vi "FipsAdjacent.vi"() -> (11 "Fips":i32[](array[numeric]))   [LabVIEW 2017] (continued)
\"Perquimans County, NC\"\t37143\n\"Perquimans County, NC\"\t37143\t\"Tyrrell County, NC\"\t37177\n\"Perquimans County, NC\"\t37143\t\"Washington County, NC\"\t37187\n\"Person County, NC\"\t37145\t\"Caswell County, NC\"\t37033\n\"Person County, NC\"\t37145\t\"Durham County, NC\"\t37063\n\"Person County, NC\"\t37145\t\"Granville County, NC\"\t37077\n\"Person County, NC\"\t37145\t\"Orange County, NC\"\t37135\n\"Person County, NC\"\t37145\t\"Person County, NC\"\t37145\n\"Person County, NC\"\t37145\t\"Halifax County, VA\"\t51083\n\"Pitt County, NC\"\t37147\t\"Beaufort County, NC\"\t37013\n\"Pitt County, NC\"\t37147\t\"Craven County, NC\"\t37049\n\"Pitt County, NC\"\t37147\t\"Edgecombe County, NC\"\t37065\n\"Pitt County, NC\"\t37147\t\"Greene County, NC\"\t37079\n\"Pitt County, NC\"\t37147\t\"Lenoir County, NC\"\t37107\n\"Pitt County, NC\"\t37147\t\"Martin County, NC\"\t37117\n\"Pitt County, NC\"\t37147\t\"Pitt County, NC\"\t37147\n\"Pitt County, NC\"\t37147\t\"Wilson County, NC\"\t37195\n\"Polk County, NC\"\t37149\t\"Henderson County, NC\"\t37089\n\"Polk County, NC\"\t37149\t\"Polk County, NC\"\t37149\n\"Polk County, NC\"\t37149\t\"Rutherford County, NC\"\t37161\n\"Polk County, NC\"\t37149\t\"Greenville County, SC\"\t45045\n\"Polk County, NC\"\t37149\t\"Spartanburg County, SC\"\t45083\n\"Randolph County, NC\"\t37151\t\"Alamance County, NC\"\t37001\n\"Randolph County, NC\"\t37151\t\"Chatham County, NC\"\t37037\n\"Randolph County, NC\"\t37151\t\"Davidson County, NC\"\t37057\n\"Randolph County, NC\"\t37151\t\"Guilford County, NC\"\t37081\n\"Randolph County, NC\"\t37151\t\"Montgomery County, NC\"\t37123\n\"Randolph County, NC\"\t37151\t\"Moore County, NC\"\t37125\n\"Randolph County, NC\"\t37151\t\"Randolph County, NC\"\t37151\n\"Richmond County, NC\"\t37153\t\"Anson County, NC\"\t37007\n\"Richmond County, NC\"\t37153\t\"Hoke County, NC\"\t37093\n\"Richmond County, NC\"\t37153\t\"Montgomery County, NC\"\t37123\n\"Richmond County, NC\"\t37153\t\"Moore County, NC\"\t37125\n\"Richmond County, NC\"\t37153\t\"Richmond County, NC\"\t37153\n\"Richmond County, NC\"\t37153\t\"Scotland County, NC\"\t37165\n\"Richmond County, NC\"\t37153\t\"Stanly County, NC\"\t37167\n\"Richmond County, NC\"\t37153\t\"Chesterfield County, SC\"\t45025\n\"Richmond County, NC\"\t37153\t\"Marlboro County, SC\"\t45069\n\"Robeson County, NC\"\t37155\t\"Bladen County, NC\"\t37017\n\"Robeson County, NC\"\t37155\t\"Columbus County, NC\"\t37047\n\"Robeson County, NC\"\t37155\t\"Cumberland County, NC\"\t37051\n\"Robeson County, NC\"\t37155\t\"Hoke County, NC\"\t37093\n\"Robeson County, NC\"\t37155\t\"Robeson County, NC\"\t37155\n\"Robeson County, NC\"\t37155\t\"Scotland County, NC\"\t37165\n\"Robeson County, NC\"\t37155\t\"Dillon County, SC\"\t45033\n\"Robeson County, NC\"\t37155\t\"Horry County, SC\"\t45051\n\"Robeson County, NC\"\t37155\t\"Marlboro County, SC\"\t45069\n\"Rockingham County, NC\"\t37157\t\"Alamance County, NC\"\t37001\n\"Rockingham County, NC\"\t37157\t\"Caswell County, NC\"\t37033\n\"Rockingham County, NC\"\t37157\t\"Forsyth County, NC\"\t37067\n\"Rockingham County, NC\"\t37157\t\"Guilford County, NC\"\t37081\n\"Rockingham County, NC\"\t37157\t\"Rockingham County, NC\"\t37157\n\"Rockingham County, NC\"\t37157\t\"Stokes County, NC\"\t37169\n\"Rockingham County, NC\"\t37157\t\"Henry County, VA\"\t51089\n\"Rockingham County, NC\"\t37157\t\"Pittsylvania County, VA\"\t51143\n\"Rowan County, NC\"\t37159\t\"Cabarrus County, NC\"\t37025\n\"Rowan County, NC\"\t37159\t\"Davidson County, NC\"\t37057\n\"Rowan County, NC\"\t37159\t\"Davie County, NC\"\t37059\n\"Rowan County, NC\"\t37159\t\"Iredell County, NC\"\t37097\n\"Rowan County, NC\"\t37159\t\"Montgomery County, NC\"\t37123\n\"Rowan County, NC\"\t37159\t\"Rowan County, NC\"\t37159\n\"Rowan County, NC\"\t37159\t\"Stanly County, NC\"\t37167\n\"Rutherford County, NC\"\t37161\t\"Buncombe County, NC\"\t37021\n\"Rutherford County, NC\"\t37161\t\"Burke County, NC\"\t37023\n\"Rutherford County, NC\"\t37161\t\"Cleveland County, NC\"\t37045\n\"Rutherford County, NC\"\t37161\t\"Henderson County, NC\"\t37089\n\"Rutherford County, NC\"\t37161\t\"McDowell County, NC\"\t37111\n\"Rutherford County, NC\"\t37161\t\"Polk County, NC\"\t37149\n\"Rutherford County, NC\"\t37161\t\"Rutherford County, NC\"\t37161\n\"Rutherford County, NC\"\t37161\t\"Cherokee County, SC\"\t45021\n\"Rutherford County, NC\"\t37161\t\"Spartanburg County, SC\"\t45083\n\"Sampson County, NC\"\t37163\t\"Bladen County, NC\"\t37017\n\"Sampson County, NC\"\t37163\t\"Cumberland County, NC\"\t37051\n\"Sampson County, NC\"\t37163\t\"Duplin County, NC\"\t37061\n\"Sampson County, NC\"\t37163\t\"Harnett County, NC\"\t37085\n\"Sampson County, NC\"\t37163\t\"Johnston County, NC\"\t37101\n\"Sampson County, NC\"\t37163\t\"Pender County, NC\"\t37141\n\"Sampson County, NC\"\t37163\t\"Sampson County, NC\"\t37163\n\"Sampson County, NC\"\t37163\t\"Wayne County, NC\"\t37191\n\"Scotland County, NC\"\t37165\t\"Hoke County, NC\"\t37093\n\"Scotland County, NC\"\t37165\t\"Moore County, NC\"\t37125\n\"Scotland County, NC\"\t37165\t\"Richmond County, NC\"\t37153\n\"Scotland County, NC\"\t37165\t\"Robeson County, NC\"\t37155\n\"Scotland County, NC\"\t37165\t\"Scotland County, NC\"\t37165\n\"Scotland County, NC\"\t37165\t\"Marlboro County, SC\"\t45069\n\"Stanly County, NC\"\t37167\t\"Anson County, NC\"\t37007\n\"Stanly County, NC\"\t37167\t\"Cabarrus County, NC\"\t37025\n\"Stanly County, NC\"\t37167\t\"Davidson County, NC\"\t37057\n\"Stanly County, NC\"\t37167\t\"Montgomery County, NC\"\t37123\n\"Stanly County, NC\"\t37167\t\"Richmond County, NC\"\t37153\n\"Stanly County, NC\"\t37167\t\"Rowan County, NC\"\t37159\n\"Stanly County, NC\"\t37167\t\"Stanly County, NC\"\t37167\n\"Stanly County, NC\"\t37167\t\"Union County, NC\"\t37179\n\"Stokes County, NC\"\t37169\t\"Forsyth County, NC\"\t37067\n\"Stokes County, NC\"\t37169\t\"Guilford County, NC\"\t37081\n\"Stokes County, NC\"\t37169\t\"Rockingham County, NC\"\t37157\n\"Stokes County, NC\"\t37169\t\"Stokes County, NC\"\t37169\n\"Stokes County, NC\"\t37169\t\"Surry County, NC\"\t37171\n\"Stokes County, NC\"\t37169\t\"Henry County, VA\"\t51089\n\"Stokes County, NC\"\t37169\t\"Patrick County, VA\"\t51141\n\"Surry County, NC\"\t37171\t\"Alleghany County, NC\"\t37005\n\"Surry County, NC\"\t37171\t\"Forsyth County, NC\"\t37067\n\"Surry County, NC\"\t37171\t\"Stokes County, NC\"\t37169\n\"Surry County, NC\"\t37171\t\"Surry County, NC\"\t37171\n\"Surry County, NC\"\t37171\t\"Wilkes County, NC\"\t37193\n\"Surry County, NC\"\t37171\t\"Yadkin County, NC\"\t37197\n\"Surry County, NC\"\t37171\t\"Carroll County, VA\"\t51035\n\"Surry County, NC\"\t37171\t\"Grayson County, VA\"\t51077\n\"Surry County, NC\"\t37171\t\"Patrick County, VA\"\t51141\n\"Swain County, NC\"\t37173\t\"Graham County, NC\"\t37075\n\"Swain County, NC\"\t37173\t\"Haywood County, NC\"\t37087\n\"Swain County, NC\"\t37173\t\"Jackson County, NC\"\t37099\n\"Swain County, NC\"\t37173\t\"Macon County, NC\"\t37113\n\"Swain County, NC\"\t37173\t\"Swain County, NC\"\t37173\n\"Swain County, NC\"\t37173\t\"Blount County, TN\"\t47009\n\"Swain County, NC\"\t37173\t\"Sevier County, TN\"\t47155\n\"Transylvania County, NC\"\t37175\t\"Haywood County, NC\"\t37087\n\"Transylvania County, NC\"\t37175\t\"Henderson County, NC\"\t37089\n\"Transylvania County, NC\"\t37175\t\"Jackson County, NC\"\t37099\n\"Transylvania County, NC\"\t37175\t\"Transylvania County, NC\"\t37175\n\"Transylvania County, NC\"\t37175\t\"Greenville County, SC\"\t45045\n\"Transylvania County, NC\"\t37175\t\"Oconee County, SC\"\t45073\n\"Transylvania County, NC\"\t37175\t\"Pickens County, SC\"\t45077\n\"Tyrrell County, NC\"\t37177\t\"Camden County, NC\"\t37029\n\"Tyrrell County, NC\"\t37177\t\"Currituck County, NC\"\t37053\n\"Tyrrell County, NC\"\t37177\t\"Dare County, NC\"\t37055\n\"Tyrrell County, NC\"\t37177\t\"Hyde County, NC\"\t37095\n\"Tyrrell County, NC\"\t37177\t\"Pasquotank County, NC\"\t37139\n\"Tyrrell County, NC\"\t37177\t\"Perquimans County, NC\"\t37143\n\"Tyrrell County, NC\"\t37177\t\"Tyrrell County, NC\"\t37177\n\"Tyrrell County, NC\"\t37177\t\"Washington County, NC\"\t37187\n\"Union County, NC\"\t37179\t\"Anson County, NC\"\t37007\n\"Union County, NC\"\t37179\t\"Cabarrus County, NC\"\t37025\n\"Union County, NC\"\t37179\t\"Mecklenburg County, NC\"\t37119\n\"Union County, NC\"\t37179\t\"Stanly County, NC\"\t37167\n\"Union County, NC\"\t37179\t\"Union County, NC\"\t37179\n\"Union County, NC\"\t37179\t\"Chesterfield County, SC\"\t45025\n\"Union County, NC\"\t37179\t\"Lancaster County, SC\"\t45057\n\"Vance County, NC\"\t37181\t\"Franklin County, NC\"\t37069\n\"Vance County, NC\"\t37181\t\"Granville County, NC\"\t37077\n\"Vance County, NC\"\t37181\t\"Vance County, NC\"\t37181\n\"Vance County, NC\"\t37181\t\"Warren County, NC\"\t37185\n\"Vance County, NC\"\t37181\t\"Mecklenburg County, VA\"\t51117\n\"Wake County, NC\"\t37183\t\"Chatham County, NC\"\t37037\n\"Wake County, NC\"\t37183\t\"Durham County, NC\"\t37063\n\"Wake County, NC\"\t37183\t\"Franklin County, NC\"\t37069\n\"Wake County, NC\"\t37183\t\"Granville County, NC\"\t37077\n\"Wake County, NC\"\t37183\t\"Harnett County, NC\"\t37085\n\"Wake County, NC\"\t37183\t\"Johnston County, NC\"\t37101\n\"Wake County, NC\"\t37183\t\"Nash County, NC\"\t37127\n\"Wake County, NC\"\t37183\t\"Wake County, NC\"\t37183\n\"Warren County, NC\"\t37185\t\"Franklin County, NC\"\t37069\n\"Warren County, NC\"\t37185\t\"Halifax County, NC\"\t37083\n\"Warren County, NC\"\t37185\t\"Nash County, NC\"\t37127\n\"Warren County, NC\"\t37185\t\"Northampton County, NC\"\t37131\n\"Warren County, NC\"\t37185\t\"Vance County, NC\"\t37181\n\"Warren County, NC\"\t37185\t\"Warren County, NC\"\t37185\n\"Warren County, NC\"\t37185\t\"Brunswick County, VA\"\t51025\n\"Warren County, NC\"\t37185\t\"Mecklenburg County, VA\"\t51117\n\"Washington County, NC\"\t37187\t\"Beaufort County, NC\"\t37013\n\"Washington County, NC\"\t37187\t\"Bertie County, NC\"\t37015\n\"Washington County, NC\"\t37187\t\"Chowan County, NC\"\t37041\n\"Washington County, NC\"\t37187\t\"Hyde County, NC\"\t37095\n\"Washington County, NC\"\t37187\t\"Martin County, NC\"\t37117\n\"Washington County, NC\"\t37187\t\"Perquimans County, NC\"\t37143\n\"Washington County, NC\"\t37187\t\"Tyrrell County, NC\"\t37177\n\"Washington County, NC\"\t37187\t\"Washington County, NC\"\t37187\n\"Watauga County, NC\"\t37189\t\"Ashe County, NC\"\t37009\n\"Watauga County, NC\"\t37189\t\"Avery County, NC\"\t37011\n\"Watauga County, NC\"\t37189\t\"Caldwell County, NC\"\t37027\n\"Watauga County, NC\"\t37189\t\"Watauga County, NC\"\t37189\n\"Watauga County, NC\"\t37189\t\"Wilkes County, NC\"\t37193\n\"Watauga County, NC\"\t37189\t\"Johnson County, TN\"\t47091\n\"Wayne County, NC\"\t37191\t\"Duplin County, NC\"\t37061\n\"Wayne County, NC\"\t37191\t\"Greene County, NC\"\t37079\n\"Wayne County, NC\"\t37191\t\"Johnston County, NC\"\t37101\n\"Wayne County, NC\"\t37191\t\"Lenoir County, NC\"\t37107\n\"Wayne County, NC\"\t37191\t\"Sampson County, NC\"\t37163\n\"Wayne County, NC\"\t37191\t\"Wayne County, NC\"\t37191\n\"Wayne County, NC\"\t37191\t\"Wilson County, NC\"\t37195\n\"Wilkes County, NC\"\t37193\t\"Alexander County, NC\"\t37003\n\"Wilkes County, NC\"\t37193\t\"Alleghany County, NC\"\t37005\n\"Wilkes County, NC\"\t37193\t\"Ashe County, NC\"\t37009\n\"Wilkes County, NC\"\t37193\t\"Caldwell County, NC\"\t37027\n\"Wilkes County, NC\"\t37193\t\"Iredell County, NC\"\t37097\n\"Wilkes County, NC\"\t37193\t\"Surry County, NC\"\t37171\n\"Wilkes County, NC\"\t37193\t\"Watauga County, NC\"\t37189\n\"Wilkes County, NC\"\t37193\t\"Wilkes County, NC\"\t37193\n\"Wilkes County, NC\"\t37193\t\"Yadkin County, NC\"\t37197\n\"Wilson County, NC\"\t37195\t\"Edgecombe County, NC\"\t37065\n\"Wilson County, NC\"\t37195\t\"Greene County, NC\"\t37079\n\"Wilson County, NC\"\t37195\t\"Johnston County, NC\"\t37101\n\"Wilson County, NC\"\t37195\t\"Nash County, NC\"\t37127\n\"Wilson County, NC\"\t37195\t\"Pitt County, NC\"\t37147\n\"Wilson County, NC\"\t37195\t\"Wayne County, NC\"\t37191\n\"Wilson County, NC\"\t37195\t\"Wilson County, NC\"\t37195\n\"Yadkin County, NC\"\t37197\t\"Davie County, NC\"\t37059\n\"Yadkin County, NC\"\t37197\t\"Forsyth County, NC\"\t37067\n\"Yadkin County, NC\"\t37197\t\"Iredell County, NC\"\t37097\n\"Yadkin County, NC\"\t37197\t\"Surry County, NC\"\t37171\n\"Yadkin County, NC\"\t37197\t\"Wilkes County, NC\"\t37193\n\"Yadkin County, NC\"\t37197\t\"Yadkin County, NC\"\t37197\n\"Yancey County, NC\"\t37199\t\"Buncombe County, NC\"\t37021\n\"Yancey County, NC\"\t37199\t\"McDowell County, NC\"\t37111\n\"Yancey County, NC\"\t37199\t\"Madison County, NC\"\t37115\n\"Yancey County, NC\"\t37199\t\"Mitchell County, NC\"\t37121\n\"Yancey County, NC\"\t37199\t\"Yancey County, NC\"\t37199\n\"Yancey County, NC\"\t37199\t\"Unicoi County, TN\"\t47171\n\"Adams County, ND\"\t38001\t\"Adams County, ND\"\t38001\n\"Adams County, ND\"\t38001\t\"Bowman County, ND\"\t38011\n\"Adams County, ND\"\t38001\t\"Grant County, ND\"\t38037\n\"Adams County, ND\"\t38001\t\"Hettinger County, ND\"\t38041\n\"Adams County, ND\"\t38001\t\"Sioux County, ND\"\t38085\n\"Adams County, ND\"\t38001\t\"Slope County, ND\"\t38087\n\"Adams County, ND\"\t38001\t\"Corson County, SD\"\t46031\n\"Adams County, ND\"\t38001\t\"Harding County, SD\"\t46063\n\"Adams County, ND\"\t38001\t\"Perkins County, SD\"\t46105\n\"Barnes County, ND\"\t38003\t\"Barnes County, ND\"\t38003\n\"Barnes County, ND\"\t38003\t\"Cass County, ND\"\t38017\n\"Barnes County, ND\"\t38003\t\"Griggs County, ND\"\t38039\n\"Barnes County, ND\"\t38003\t\"LaMoure County, ND\"\t38045\n\"Barnes County, ND\"\t38003\t\"Ransom County, ND\"\t38073\n\"Barnes County, ND\"\t38003\t\"Steele County, ND\"\t38091\n\"Barnes County, ND\"\t38003\t\"Stutsman County, ND\"\t38093\n\"Benson County, ND\"\t38005\t\"Benson County, ND\"\t38005\n\"Benson County, ND\"\t38005\t\"Eddy County, ND\"\t38027\n\"Benson County, ND\"\t38005\t\"Nelson County, ND\"\t38063\n\"Benson County, ND\"\t38005\t\"Pierce County, ND\"\t38069\n\"Benson County, ND\"\t38005\t\"Ramsey County, ND\"\t38071\n\"Benson County, ND\"\t38005\t\"Towner County, ND\"\t38095\n\"Benson County, ND\"\t38005\t\"Wells County, ND\"\t38103\n\"Billings County, ND\"\t38007\t\"Billings County, ND\"\t38007\n\"Billings County, ND\"\t38007\t\"Dunn County, ND\"\t38025\n\"Billings County, ND\"\t38007\t\"Golden Valley County, ND\"\t38033\n\"Billings County, ND\"\t38007\t\"McKenzie County, ND\"\t38053\n\"Billings County, ND\"\t38007\t\"Slope County, ND\"\t38087\n\"Billings County, ND\"\t38007\t\"Stark County, ND\"\t38089\n\"Bottineau County, ND\"\t38009\t\"Bottineau County, ND\"\t38009\n\"Bottineau County, ND\"\t38009\t\"McHenry County, ND\"\t38049\n\"Bottineau County, ND\"\t38009\t\"Pierce County, ND\"\t38069\n\"Bottineau County, ND\"\t38009\t\"Renville County, ND\"\t38075\n\"Bottineau County, ND\"\t38009\t\"Rolette County, ND\"\t38079\n\"Bowman County, ND\"\t38011\t\"Fallon County, MT\"\t30025\n\"Bowman County, ND\"\t38011\t\"Adams County, ND\"\t38001\n\"Bowman County, ND\"\t38011\t\"Bowman County, ND\"\t38011\n\"Bowman County, ND\"\t38011\t\"Slope County, ND\"\t38087\n\"Bowman County, ND\"\t38011\t\"Harding County, SD\"\t46063\n\"Burke County, ND\"\t38013\t\"Burke County, ND\"\t38013\n\"Burke County, ND\"\t38013\t\"Divide County, ND\"\t38023\n\"Burke County, ND\"\t38013\t\"Mountrail County, ND\"\t38061\n\"Burke County, ND\"\t38013\t\"Renville County, ND\"\t38075\n\"Burke County, ND\"\t38013\t\"Ward County, ND\"\t38101\n\"Burke County, ND\"\t38013\t\"Williams County, ND\"\t38105\n\"Burleigh County, ND\"\t38015\t\"Burleigh County, ND\"\t38015\n\"Burleigh County, ND\"\t38015\t\"Emmons County, ND\"\t38029\n\"Burleigh County, ND\"\t38015\t\"Kidder County, ND\"\t38043\n\"Burleigh County, ND\"\t38015\t\"McLean County, ND\"\t38055\n\"Burleigh County, ND\"\t38015\t\"Morton County, ND\"\t38059\n\"Burleigh County, ND\"\t38015\t\"Oliver County, ND\"\t38065\n\"Burleigh County, ND\"\t38015\t\"Sheridan County, ND\"\t38083\n\"Cass County, ND\"\t38017\t\"Clay County, MN\"\t27027\n\"Cass County, ND\"\t38017\t\"Norman County, MN\"\t27107\n\"Cass County, ND\"\t38017\t\"Barnes County, ND\"\t38003\n\"Cass County, ND\"\t38017\t\"Cass County, ND\"\t38017\n\"Cass County, ND\"\t38017\t\"Ransom County, ND\"\t38073\n\"Cass County, ND\"\t38017\t\"Richland County, ND\"\t38077\n\"Cass County, ND\"\t38017\t\"Steele County, ND\"\t38091\n\"Cass County, ND\"\t38017\t\"Traill County, ND\"\t38097\n\"Cavalier County, ND\"\t38019\t\"Cavalier County, ND\"\t38019\n\"Cavalier County, ND\"\t38019\t\"Pembina County, ND\"\t38067\n\"Cavalier County, ND\"\t38019\t\"Ramsey County, ND\"\t38071\n\"Cavalier County, ND\"\t38019\t\"Towner County, ND\"\t38095\n\"Cavalier County, ND\"\t38019\t\"Walsh County, ND\"\t38099\n\"Dickey County, ND\"\t38021\t\"Dickey County, ND\"\t38021\n\"Dickey County, ND\"\t38021\t\"LaMoure County, ND\"\t38045\n\"Dickey County, ND\"\t38021\t\"McIntosh County, ND\"\t38051\n\"Dickey County, ND\"\t38021\t\"Ransom County, ND\"\t38073\n\"Dickey County, ND\"\t38021\t\"Sargent County, ND\"\t38081\n\"Dickey County, ND\"\t38021\t\"Brown County, SD\"\t46013\n\"Dickey County, ND\"\t38021\t\"McPherson County, SD\"\t46089\n\"Divide County, ND\"\t38023\t\"Sheridan County, MT\"\t30091\n\"Divide County, ND\"\t38023\t\"Burke County, ND\"\t38013\n\"Divide County, ND\"\t38023\t\"Divide County, ND\"\t38023\n\"Divide County, ND\"\t38023\t\"Williams County, ND\"\t38105\n\"Dunn County, ND\"\t38025\t\"Billings County, ND\"\t38007\n\"Dunn County, ND\"\t38025\t\"Dunn County, ND\"\t38025\n\"Dunn County, ND\"\t38025\t\"McKenzie County, ND\"\t38053\n\"Dunn County, ND\"\t38025\t\"McLean County, ND\"\t38055\n\"Dunn County, ND\"\t38025\t\"Mercer County, ND\"\t38057\n\"Dunn County, ND\"\t38025\t\"Mountrail County, ND\"\t38061\n\"Dunn County, ND\"\t38025\t\"Stark County, ND\"\t38089\n\"Eddy County, ND\"\t38027\t\"Benson County, ND\"\t38005\n\"Eddy County, ND\"\t38027\t\"Eddy County, ND\"\t38027\n\"Eddy County, ND\"\t38027\t\"Foster County, ND\"\t38031\n\"Eddy County, ND\"\t38027\t\"Griggs County, ND\"\t38039\n\"Eddy County, ND\"\t38027\t\"Nelson County, ND\"\t38063\n\"Eddy County, ND\"\t38027\t\"Wells County, ND\"\t38103\n\"Emmons County, ND\"\t38029\t\"Burleigh County, ND\"\t38015\n\"Emmons County, ND\"\t38029\t\"Emmons County, ND\"\t38029\n\"Emmons County, ND\"\t38029\t\"Kidder County, ND\"\t38043\n\"Emmons County, ND\"\t38029\t\"Logan County, ND\"\t38047\n\"Emmons County, ND\"\t38029\t\"McIntosh County, ND\"\t38051\n\"Emmons County, ND\"\t38029\t\"Morton County, ND\"\t38059\n\"Emmons County, ND\"\t38029\t\"Sioux County, ND\"\t38085\n\"Emmons County, ND\"\t38029\t\"Campbell County, SD\"\t46021\n\"Emmons County, ND\"\t38029\t\"Corson County, SD\"\t46031\n\"Foster County, ND\"\t38031\t\"Eddy County, ND\"\t38027\n\"Foster County, ND\"\t38031\t\"Foster County, ND\"\t38031\n\"Foster County, ND\"\t38031\t\"Griggs County, ND\"\t38039\n\"Foster County, ND\"\t38031\t\"Stutsman County, ND\"\t38093\n\"Foster County, ND\"\t38031\t\"Wells County, ND\"\t38103\n\"Golden Valley County, ND\"\t38033\t\"Fallon County, MT\"\t30025\n\"Golden Valley County, ND\"\t38033\t\"Wibaux County, MT\"\t30109\n\"Golden Valley County, ND\"\t38033\t\"Billings County, ND\"\t38007\n\"Golden Valley County, ND\"\t38033\t\"Golden Valley County, ND\"\t38033\n\"Golden Valley County, ND\"\t38033\t\"McKenzie County, ND\"\t38053\n\"Golden Valley County, ND\"\t38033\t\"Slope County, ND\"\t38087\n\"Grand Forks County, ND\"\t38035\t\"Marshall County, MN\"\t27089\n\"Grand Forks County, ND\"\t38035\t\"Polk County, MN\"\t27119\n\"Grand Forks County, ND\"\t38035\t\"Grand Forks County, ND\"\t38035\n\"Grand Forks County, ND\"\t38035\t\"Nelson County, ND\"\t38063\n\"Grand Forks County, ND\"\t38035\t\"Steele County, ND\"\t38091\n\"Grand Forks County, ND\"\t38035\t\"Traill County, ND\"\t38097\n\"Grand Forks County, ND\"\t38035\t\"Walsh County, ND\"\t38099\n\"Grant County, ND\"\t38037\t\"Adams County, ND\"\t38001\n\"Grant County, ND\"\t38037\t\"Grant County, ND\"\t38037\n\"Grant County, ND\"\t38037\t\"Hettinger County, ND\"\t38041\n\"Grant County, ND\"\t38037\t\"Morton County, ND\"\t38059\n\"Grant County, ND\"\t38037\t\"Sioux County, ND\"\t38085\n\"Grant County, ND\"\t38037\t\"Stark County, ND\"\t38089\n\"Griggs County, ND\"\t38039\t\"Barnes County, ND\"\t38003\n\"Griggs County, ND\"\t38039\t\"Eddy County, ND\"\t38027\n\"Griggs County, ND\"\t38039\t\"Foster County, ND\"\t38031\n\"Griggs County, ND\"\t38039\t\"Griggs County, ND\"\t38039\n\"Griggs County, ND\"\t38039\t\"Nelson County, ND\"\t38063\n\"Griggs County, ND\"\t38039\t\"Steele County, ND\"\t38091\n\"Griggs County, ND\"\t38039\t\"Stutsman County, ND\"\t38093\n\"Hettinger County, ND\"\t38041\t\"Adams County, ND\"\t38001\n\"Hettinger County, ND\"\t38041\t\"Grant County, ND\"\t38037\n\"Hettinger County, ND\"\t38041\t\"Hettinger County, ND\"\t38041\n\"Hettinger County, ND\"\t38041\t\"Slope County, ND\"\t38087\n\"Hettinger County, ND\"\t38041\t\"Stark County, ND\"\t38089\n\"Kidder County, ND\"\t38043\t\"Burleigh County, ND\"\t38015\n\"Kidder County, ND\"\t38043\t\"Emmons County, ND\"\t38029\n\"Kidder County, ND\"\t38043\t\"Kidder County, ND\"\t38043\n\"Kidder County, ND\"\t38043\t\"Logan County, ND\"\t38047\n\"Kidder County, ND\"\t38043\t\"Sheridan County, ND\"\t38083\n\"Kidder County, ND\"\t38043\t\"Stutsman County, ND\"\t38093\n\"Kidder County, ND\"\t38043\t\"Wells County, ND\"\t38103\n\"LaMoure County, ND\"\t38045\t\"Barnes County, ND\"\t38003\n\"LaMoure County, ND\"\t38045\t\"Dickey County, ND\"\t38021\n\"LaMoure County, ND\"\t38045\t\"LaMoure County, ND\"\t38045\n\"LaMoure County, ND\"\t38045\t\"Logan County, ND\"\t38047\n\"LaMoure County, ND\"\t38045\t\"McIntosh County, ND\"\t38051\n\"LaMoure County, ND\"\t38045\t\"Ransom County, ND\"\t38073\n\"LaMoure County, ND\"\t38045\t\"Stutsman County, ND\"\t38093\n\"Logan County, ND\"\t38047\t\"Emmons County, ND\"\t38029\n\"Logan County, ND\"\t38047\t\"Kidder County, ND\"\t38043\n\"Logan County, ND\"\t38047\t\"LaMoure County, ND\"\t38045\n\"Logan County, ND\"\t38047\t\"Logan County, ND\"\t38047\n\"Logan County, ND\"\t38047\t\"McIntosh County, ND\"\t38051\n\"Logan County, ND\"\t38047\t\"Stutsman County, ND\"\t38093\n\"McHenry County, ND\"\t38049\t\"Bottineau County, ND\"\t38009\n\"McHenry County, ND\"\t38049\t\"McHenry County, ND\"\t38049\n\"McHenry County, ND\"\t38049\t\"McLean County, ND\"\t38055\n\"McHenry County, ND\"\t38049\t\"Pierce County, ND\"\t38069\n\"McHenry County, ND\"\t38049\t\"Renville County, ND\"\t38075\n\"McHenry County, ND\"\t38049\t\"Sheridan County, ND\"\t38083\n\"McHenry County, ND\"\t38049\t\"Ward County, ND\"\t38101\n\"McIntosh County, ND\"\t38051\t\"Dickey County, ND\"\t38021\n\"McIntosh County, ND\"\t38051\t\"Emmons County, ND\"\t38029\n\"McIntosh County, ND\"\t38051\t\"LaMoure County, ND\"\t38045\n\"McIntosh County, ND\"\t38051\t\"Logan County, ND\"\t38047\n\"McIntosh County, ND\"\t38051\t\"McIntosh County, ND\"\t38051\n\"McIntosh County, ND\"\t38051\t\"Campbell County, SD\"\t46021\n\"McIntosh County, ND\"\t38051\t\"McPherson County, SD\"\t46089\n\"McKenzie County, ND\"\t38053\t\"Richland County, MT\"\t30083\n\"McKenzie County, ND\"\t38053\t\"Roosevelt County, MT\"\t30085\n\"McKenzie County, ND\"\t38053\t\"Wibaux County, MT\"\t30109\n\"McKenzie County, ND\"\t38053\t\"Billings County, ND\"\t38007\n\"McKenzie County, ND\"\t38053\t\"Dunn County, ND\"\t38025\n\"McKenzie County, ND\"\t38053\t\"Golden Valley County, ND\"\t38033\n\"McKenzie County, ND\"\t38053\t\"McKenzie County, ND\"\t38053\n\"McKenzie County, ND\"\t38053\t\"Mountrail County, ND\"\t38061\n\"McKenzie County, ND\"\t38053\t\"Williams County, ND\"\t38105\n\"McLean County, ND\"\t38055\t\"Burleigh County, ND\"\t38015\n\"McLean County, ND\"\t38055\t\"Dunn County, ND\"\t38025\n\"McLean County, ND\"\t38055\t\"McHenry County, ND\"\t38049\n\"McLean County, ND\"\t38055\t\"McLean County, ND\"\t38055\n\"McLean County, ND\"\t38055\t\"Mercer County, ND\"\t38057\n\"McLean County, ND\"\t38055\t\"Mountrail County, ND\"\t38061\n\"McLean County, ND\"\t38055\t\"Oliver County, ND\"\t38065\n\"McLean County, ND\"\t38055\t\"Sheridan County, ND\"\t38083\n\"McLean County, ND\"\t38055\t\"Ward County, ND\"\t38101\n\"Mercer County, ND\"\t38057\t\"Dunn County, ND\"\t38025\n\"Mercer County, ND\"\t38057\t\"McLean County, ND\"\t38055\n\"Mercer County, ND\"\t38057\t\"Mercer County, ND\"\t38057\n\"Mercer County, ND\"\t38057\t\"Morton County, ND\"\t38059\n\"Mercer County, ND\"\t38057\t\"Oliver County, ND\"\t38065\n\"Mercer County, ND\"\t38057\t\"Stark County, ND\"\t38089\n\"Morton County, ND\"\t38059\t\"Burleigh County, ND\"\t38015\n\"Morton County, ND\"\t38059\t\"Emmons County, ND\"\t38029\n\"Morton County, ND\"\t38059\t\"Grant County, ND\"\t38037\n\"Morton County, ND\"\t38059\t\"Mercer County, ND\"\t38057\n\"Morton County, ND\"\t38059\t\"Morton County, ND\"\t38059\n\"Morton County, ND\"\t38059\t\"Oliver County, ND\"\t38065\n\"Morton County, ND\"\t38059\t\"Sioux County, ND\"\t38085\n\"Morton County, ND\"\t38059\t\"Stark County, ND\"\t38089\n\"Mountrail County, ND\"\t38061\t\"Burke County, ND\"\t38013\n\"Mountrail County, ND\"\t38061\t\"Dunn County, ND\"\t38025\n\"Mountrail County, ND\"\t38061\t\"McKenzie County, ND\"\t38053\n\"Mountrail County, ND\"\t38061\t\"McLean County, ND\"\t38055\n\"Mountrail County, ND\"\t38061\t\"Mountrail County, ND\"\t38061\n\"Mountrail County, ND\"\t38061\t\"Ward County, ND\"\t38101\n\"Mountrail County, ND\"\t38061\t\"Williams County, ND\"\t38105\n\"Nelson County, ND\"\t38063\t\"Benson County, ND\"\t38005\n\"Nelson County, ND\"\t38063\t\"Eddy County, ND\"\t38027\n\"Nelson County, ND\"\t38063\t\"Grand Forks County, ND\"\t38035\n\"Nelson County, ND\"\t38063\t\"Griggs County, ND\"\t38039\n\"Nelson County, ND\"\t38063\t\"Nelson County, ND\"\t38063\n\"Nelson County, ND\"\t38063\t\"Ramsey County, ND\"\t38071\n\"Nelson County, ND\"\t38063\t\"Steele County, ND\"\t38091\n\"Nelson County, ND\"\t38063\t\"Walsh County, ND\"\t38099\n\"Oliver County, ND\"\t38065\t\"Burleigh County, ND\"\t38015\n\"Oliver County, ND\"\t38065\t\"McLean County, ND\"\t38055\n\"Oliver County, ND\"\t38065\t\"Mercer County, ND\"\t38057\n\"Oliver County, ND\"\t38065\t\"Morton County, ND\"\t38059\n\"Oliver County, ND\"\t38065\t\"Oliver County, ND\"\t38065\n\"Pembina County, ND\"\t38067\t\"Kittson County, MN\"\t27069\n\"Pembina County, ND\"\t38067\t\"Marshall County, MN\"\t27089\n\"Pembina County, ND\"\t38067\t\"Cavalier County, ND\"\t38019\n\"Pembina County, ND\"\t38067\t\"Pembina County, ND\"\t38067\n\"Pembina County, ND\"\t38067\t\"Walsh County, ND\"\t38099\n\"Pierce County, ND\"\t38069\t\"Benson County, ND\"\t38005\n\"Pierce County, ND\"\t38069\t\"Bottineau County, ND\"\t38009\n\"Pierce County, ND\"\t38069\t\"McHenry County, ND\"\t38049\n\"Pierce County, ND\"\t38069\t\"Pierce County, ND\"\t38069\n\"Pierce County, ND\"\t38069\t\"Rolette County, ND\"\t38079\n\"Pierce County, ND\"\t38069\t\"Sheridan County, ND\"\t38083\n\"Pierce County, ND\"\t38069\t\"Towner County, ND\"\t38095\n\"Pierce County, ND\"\t38069\t\"Wells County, ND\"\t38103\n\"Ramsey County, ND\"\t38071\t\"Benson County, ND\"\t38005\n\"Ramsey County, ND\"\t38071\t\"Cavalier County, ND\"\t38019\n\"Ramsey County, ND\"\t38071\t\"Nelson County, ND\"\t38063\n\"Ramsey County, ND\"\t38071\t\"Ramsey County, ND\"\t38071\n\"Ramsey County, ND\"\t38071\t\"Towner County, ND\"\t38095\n\"Ramsey County, ND\"\t38071\t\"Walsh County, ND\"\t38099\n\"Ransom County, ND\"\t38073\t\"Barnes County, ND\"\t38003\n\"Ransom County, ND\"\t38073\t\"Cass County, ND\"\t38017\n\"Ransom County, ND\"\t38073\t\"Dickey County, ND\"\t38021\n\"Ransom County, ND\"\t38073\t\"LaMoure County, ND\"\t38045\n\"Ransom County, ND\"\t38073\t\"Ransom County, ND\"\t38073\n\"Ransom County, ND\"\t38073\t\"Richland County, ND\"\t38077\n\"Ransom County, ND\"\t38073\t\"Sargent County, ND\"\t38081\n\"Renville County, ND\"\t38075\t\"Bottineau County, ND\"\t38009\n\"Renville County, ND\"\t38075\t\"Burke County, ND\"\t38013\n\"Renville County, ND\"\t38075\t\"McHenry County, ND\"\t38049\n\"Renville County, ND\"\t38075\t\"Renville County, ND\"\t38075\n\"Renville County, ND\"\t38075\t\"Ward County, ND\"\t38101\n\"Richland County, ND\"\t38077\t\"Clay County, MN\"\t27027\n\"Richland County, ND\"\t38077\t\"Traverse County, MN\"\t27155\n\"Richland County, ND\"\t38077\t\"Wilkin County, MN\"\t27167\n\"Richland County, ND\"\t38077\t\"Cass County, ND\"\t38017\n\"Richland County, ND\"\t38077\t\"Ransom County, ND\"\t38073\n\"Richland County, ND\"\t38077\t\"Richland County, ND\"\t38077\n\"Richland County, ND\"\t38077\t\"Sargent County, ND\"\t38081\n\"Richland County, ND\"\t38077\t\"Marshall County, SD\"\t46091\n\"Richland County, ND\"\t38077\t\"Roberts County, SD\"\t46109\n\"Rolette County, ND\"\t38079\t\"Bottineau County, ND\"\t38009\n\"Rolette County, ND\"\t38079\t\"Pierce County, ND\"\t38069\n\"Rolette County, ND\"\t38079\t\"Rolette County, ND\"\t38079\n\"Rolette County, ND\"\t38079\t\"Towner County, ND\"\t38095\n\"Sargent County, ND\"\t38081\t\"Dickey County, ND\"\t38021\n\"Sargent County, ND\"\t38081\t\"Ransom County, ND\"\t38073\n\"Sargent County, ND\"\t38081\t\"Richland County, ND\"\t38077\n\"Sargent County, ND\"\t38081\t\"Sargent County, ND\"\t38081\n\"Sargent County, ND\"\t38081\t\"Brown County, SD\"\t46013\n\"Sargent County, ND\"\t38081\t\"Marshall County, SD\"\t46091\n\"Sargent County, ND\"\t38081\t\"Roberts County, SD\"\t46109\n\"Sheridan County, ND\"\t38083\t\"Burleigh County, ND\"\t38015\n\"Sheridan County, ND\"\t38083\t\"Kidder County, ND\"\t38043\n\"Sheridan County, ND\"\t38083\t\"McHenry County, ND\"\t38049\n\"Sheridan County, ND\"\t38083\t\"McLean County, ND\"\t38055\n\"Sheridan County, ND\"\t38083\t\"Pierce County, ND\"\t38069\n\"Sheridan County, ND\"\t38083\t\"Sheridan County, ND\"\t38083\n\"Sheridan County, ND\"\t38083\t\"Wells County, ND\"\t38103\n\"Sioux County, ND\"\t38085\t\"Adams County, ND\"\t38001\n\"Sioux County, ND\"\t38085\t\"Emmons County, ND\"\t38029\n\"Sioux County, ND\"\t38085\t\"Grant County, ND\"\t38037\n\"Sioux County, ND\"\t38085\t\"Morton County, ND\"\t38059\n\"Sioux County, ND\"\t38085\t\"Sioux County, ND\"\t38085\n\"Sioux County, ND\"\t38085\t\"Corson County, SD\"\t46031\n\"Slope County, ND\"\t38087\t\"Fallon County, MT\"\t30025\n\"Slope County, ND\"\t38087\t\"Adams County, ND\"\t38001\n\"Slope County, ND\"\t38087\t\"Billings County, ND\"\t38007\n\"Slope County, ND\"\t38087\t\"Bowman County, ND\"\t38011\n\"Slope County, ND\"\t38087\t\"Golden Valley County, ND\"\t38033\n\"Slope County, ND\"\t38087\t\"Hettinger County, ND\"\t38041\n\"Slope County, ND\"\t38087\t\"Slope County, ND\"\t38087\n\"Slope County, ND\"\t38087\t\"Stark County, ND\"\t38089\n\"Stark County, ND\"\t38089\t\"Billings County, ND\"\t38007\n\"Stark County, ND\"\t38089\t\"Dunn County, ND\"\t38025\n\"Stark County, ND\"\t38089\t\"Grant County, ND\"\t38037\n\"Stark County, ND\"\t38089\t\"Hettinger County, ND\"\t38041\n\"Stark County, ND\"\t38089\t\"Mercer County, ND\"\t38057\n\"Stark County, ND\"\t38089\t\"Morton County, ND\"\t38059\n\"Stark County, ND\"\t38089\t\"Slope County, ND\"\t38087\n\"Stark County, ND\"\t38089\t\"Stark County, ND\"\t38089\n\"Steele County, ND\"\t38091\t\"Barnes County, ND\"\t38003\n\"Steele County, ND\"\t38091\t\"Cass County, ND\"\t38017\n\"Steele County, ND\"\t38091\t\"Grand Forks County, ND\"\t38035\n\"Steele County, ND\"\t38091\t\"Griggs County, ND\"\t38039\n\"Steele County, ND\"\t38091\t\"Nelson County, ND\"\t38063\n\"Steele County, ND\"\t38091\t\"Steele County, ND\"\t38091\n\"Steele County, ND\"\t38091\t\"Traill County, ND\"\t38097\n\"Stutsman County, ND\"\t38093\t\"Barnes County, ND\"\t38003\n\"Stutsman County, ND\"\t38093\t\"Foster County, ND\"\t38031\n\"Stutsman County, ND\"\t38093\t\"Griggs County, ND\"\t38039\n\"Stutsman County, ND\"\t38093\t\"Kidder County, ND\"\t38043\n\"Stutsman County, ND\"\t38093\t\"LaMoure County, ND\"\t38045\n\"Stutsman County, ND\"\t38093\t\"Logan County, ND\"\t38047\n\"Stutsman County, ND\"\t38093\t\"Stutsman County, ND\"\t38093\n\"Stutsman County, ND\"\t38093\t\"Wells County, ND\"\t38103\n\"Towner County, ND\"\t38095\t\"Benson County, ND\"\t38005\n\"Towner County, ND\"\t38095\t\"Cavalier County, ND\"\t38019\n\"Towner County, ND\"\t38095\t\"Pierce County, ND\"\t38069\n\"Towner County, ND\"\t38095\t\"Ramsey County, ND\"\t38071\n\"Towner County, ND\"\t38095\t\"Rolette County, ND\"\t38079\n\"Towner County, ND\"\t38095\t\"Towner County, ND\"\t38095\n\"Traill County, ND\"\t38097\t\"Norman County, MN\"\t27107\n\"Traill County, ND\"\t38097\t\"Polk County, MN\"\t27119\n\"Traill County, ND\"\t38097\t\"Cass County, ND\"\t38017\n\"Traill County, ND\"\t38097\t\"Grand Forks County, ND\"\t38035\n\"Traill County, ND\"\t38097\t\"Steele County, ND\"\t38091\n\"Traill County, ND\"\t38097\t\"Traill County, ND\"\t38097\n\"Walsh County, ND\"\t38099\t\"Marshall County, MN\"\t27089\n\"Walsh County, ND\"\t38099\t\"Cavalier County, ND\"\t38019\n\"Walsh County, ND\"\t38099\t\"Grand Forks County, ND\"\t38035\n\"Walsh County, ND\"\t38099\t\"Nelson County, ND\"\t38063\n\"Walsh County, ND\"\t38099\t\"Pembina County, ND\"\t38067\n\"Walsh County, ND\"\t38099\t\"Ramsey County, ND\"\t38071\n\"Walsh County, ND\"\t38099\t\"Walsh County, ND\"\t38099\n\"Ward County, ND\"\t38101\t\"Burke County, ND\"\t38013\n\"Ward County, ND\"\t38101\t\"McHenry County, ND\"\t38049\n\"Ward County, ND\"\t38101\t\"McLean County, ND\"\t38055\n\"Ward County, ND\"\t38101\t\"Mountrail County, ND\"\t38061\n\"Ward County, ND\"\t38101\t\"Renville County, ND\"\t38075\n\"Ward County, ND\"\t38101\t\"Ward County, ND\"\t38101\n\"Wells County, ND\"\t38103\t\"Benson County, ND\"\t38005\n\"Wells County, ND\"\t38103\t\"Eddy County, ND\"\t38027\n\"Wells County, ND\"\t38103\t\"Foster County, ND\"\t38031\n\"Wells County, ND\"\t38103\t\"Kidder County, ND\"\t38043\n\"Wells County, ND\"\t38103\t\"Pierce County, ND\"\t38069\n\"Wells County, ND\"\t38103\t\"Sheridan County, ND\"\t38083\n\"Wells County, ND\"\t38103\t\"Stutsman County, ND\"\t38093\n\"Wells County, ND\"\t38103\t\"Wells County, ND\"\t38103\n\"Williams County, ND\"\t38105\t\"Richland County, MT\"\t30083\n\"Williams County, ND\"\t38105\t\"Roosevelt County, MT\"\t30085\n\"Williams County, ND\"\t38105\t\"Sheridan County, MT\"\t30091\n\"Williams County, ND\"\t38105\t\"Burke County, ND\"\t38013\n\"Williams County, ND\"\t38105\t\"Divide County, ND\"\t38023\n\"Williams County, ND\"\t38105\t\"McKenzie County, ND\"\t38053\n\"Williams County, ND\"\t38105\t\"Mountrail County, ND\"\t38061\n\"Williams County, ND\"\t38105\t\"Williams County, ND\"\t38105\n\"Adams County, OH\"\t39001\t\"Lewis County, KY\"\t21135\n\"Adams County, OH\"\t39001\t\"Mason County, KY\"\t21161\n\"Adams County, OH\"\t39001\t\"Adams County, OH\"\t39001\n\"Adams County, OH\"\t39001\t\"Brown County, OH\"\t39015\n\"Adams County, OH\"\t39001\t\"Highland County, OH\"\t39071\n\"Adams County, OH\"\t39001\t\"Pike County, OH\"\t39131\n\"Adams County, OH\"\t39001\t\"Scioto County, OH\"\t39145\n\"Allen County, OH\"\t39003\t\"Allen County, OH\"\t39003\n\"Allen County, OH\"\t39003\t\"Auglaize County, OH\"\t39011\n\"Allen County, OH\"\t39003\t\"Hancock County, OH\"\t39063\n\"Allen County, OH\"\t39003\t\"Hardin County, OH\"\t39065\n\"Allen County, OH\"\t39003\t\"Putnam County, OH\"\t39137\n\"Allen County, OH\"\t39003\t\"Van Wert County, OH\"\t39161\n\"Ashland County, OH\"\t39005\t\"Ashland County, OH\"\t39005\n\"Ashland County, OH\"\t39005\t\"Holmes County, OH\"\t39075\n\"Ashland County, OH\"\t39005\t\"Huron County, OH\"\t39077\n\"Ashland County, OH\"\t39005\t\"Knox County, OH\"\t39083\n\"Ashland County, OH\"\t39005\t\"Lorain County, OH\"\t39093\n\"Ashland County, OH\"\t39005\t\"Medina County, OH\"\t39103\n\"Ashland County, OH\"\t39005\t\"Richland County, OH\"\t39139\n\"Ashland County, OH\"\t39005\t\"Wayne County, OH\"\t39169\n\"Ashtabula County, OH\"\t39007\t\"Ashtabula County, OH\"\t39007\n\"Ashtabula County, OH\"\t39007\t\"Geauga County, OH\"\t39055\n\"Ashtabula County, OH\"\t39007\t\"Lake County, OH\"\t39085\n\"Ashtabula County, OH\"\t39007\t\"Trumbull County, OH\"\t39155\n\"Ashtabula County, OH\"\t39007\t\"Crawford County, PA\"\t42039\n\"Ashtabula County, OH\"\t39007\t\"Erie County, PA\"\t42049\n\"Athens County, OH\"\t39009\t\"Athens County, OH\"\t39009\n\"Athens County, OH\"\t39009\t\"Hocking County, OH\"\t39073\n\"Athens County, OH\"\t39009\t\"Meigs County, OH\"\t39105\n\"Athens County, OH\"\t39009\t\"Morgan County, OH\"\t39115\n\"Athens County, OH\"\t39009\t\"Perry County, OH\"\t39127\n\"Athens County, OH\"\t39009\t\"Vinton County, OH\"\t39163\n\"Athens County, OH\"\t39009\t\"Washington County, OH\"\t39167\n\"Athens County, OH\"\t39009\t\"Wood County, WV\"\t54107\n\"Auglaize County, OH\"\t39011\t\"Allen County, OH\"\t39003\n\"Auglaize County, OH\"\t39011\t\"Auglaize County, OH\"\t39011\n\"Auglaize County, OH\"\t39011\t\"Hardin County, OH\"\t39065\n\"Auglaize County, OH\"\t39011\t\"Logan County, OH\"\t39091\n\"Auglaize County, OH\"\t39011\t\"Mercer County, OH\"\t39107\n\"Auglaize County, OH\"\t39011\t\"Shelby County, OH\"\t39149\n\"Auglaize County, OH\"\t39011\t\"Van Wert County, OH\"\t39161\n\"Belmont County, OH\"\t39013\t\"Belmont County, OH\"\t39013\n\"Belmont County, OH\"\t39013\t\"Guernsey County, OH\"\t39059\n\"Belmont County, OH\"\t39013\t\"Harrison County, OH\"\t39067\n\"Belmont County, OH\"\t39013\t\"Jefferson County, OH\"\t39081\n\"Belmont County, OH\"\t39013\t\"Monroe County, OH\"\t39111\n\"Belmont County, OH\"\t39013\t\"Noble County, OH\"\t39121\n\"Belmont County, OH\"\t39013\t\"Marshall County, WV\"\t54051\n\"Belmont County, OH\"\t39013\t\"Ohio County, WV\"\t54069\n\"Brown County, OH\"\t39015\t\"Bracken County, KY\"\t21023\n\"Brown County, OH\"\t39015\t\"Mason County, KY\"\t21161\n\"Brown County, OH\"\t39015\t\"Adams County, OH\"\t39001\n\"Brown County, OH\"\t39015\t\"Brown County, OH\"\t39015\n\"Brown County, OH\"\t39015\t\"Clermont County, OH\"\t39025\n\"Brown County, OH\"\t39015\t\"Clinton County, OH\"\t39027\n\"Brown County, OH\"\t39015\t\"Highland County, OH\"\t39071\n\"Butler County, OH\"\t39017\t\"Dearborn County, IN\"\t18029\n\"Butler County, OH\"\t39017\t\"Franklin County, IN\"\t18047\n\"Butler County, OH\"\t39017\t\"Union County, IN\"\t18161\n\"Butler County, OH\"\t39017\t\"Butler County, OH\"\t39017\n\"Butler County, OH\"\t39017\t\"Hamilton County, OH\"\t39061\n\"Butler County, OH\"\t39017\t\"Montgomery County, OH\"\t39113\n\"Butler County, OH\"\t39017\t\"Preble County, OH\"\t39135\n\"Butler County, OH\"\t39017\t\"Warren County, OH\"\t39165\n\"Carroll County, OH\"\t39019\t\"Carroll County, OH\"\t39019\n\"Carroll County, OH\"\t39019\t\"Columbiana County, OH\"\t39029\n\"Carroll County, OH\"\t39019\t\"Harrison County, OH\"\t39067\n\"Carroll County, OH\"\t39019\t\"Jefferson County, OH\"\t39081\n\"Carroll County, OH\"\t39019\t\"Stark County, OH\"\t39151\n\"Carroll County, OH\"\t39019\t\"Tuscarawas County, OH\"\t39157\n\"Champaign County, OH\"\t39021\t\"Champaign County, OH\"\t39021\n\"Champaign County, OH\"\t39021\t\"Clark County, OH\"\t39023\n\"Champaign County, OH\"\t39021\t\"Logan County, OH\"\t39091\n\"Champaign County, OH\"\t39021\t\"Madison County, OH\"\t39097\n\"Champaign County, OH\"\t39021\t\"Miami County, OH\"\t39109\n\"Champaign County, OH\"\t39021\t\"Shelby County, OH\"\t39149\n\"Champaign County, OH\"\t39021\t\"Union County, OH\"\t39159\n\"Clark County, OH\"\t39023\t\"Champaign County, OH\"\t39021\n\"Clark County, OH\"\t39023\t\"Clark County, OH\"\t39023\n\"Clark County, OH\"\t39023\t\"Greene County, OH\"\t39057\n\"Clark County, OH\"\t39023\t\"Madison County, OH\"\t39097\n\"Clark County, OH\"\t39023\t\"Miami County, OH\"\t39109\n\"Clark County, OH\"\t39023\t\"Montgomery County, OH\"\t39113\n\"Clermont County, OH\"\t39025\t\"Bracken County, KY\"\t21023\n\"Clermont County, OH\"\t39025\t\"Campbell County, KY\"\t21037\n\"Clermont County, OH\"\t39025\t\"Pendleton County, KY\"\t21191\n\"Clermont County, OH\"\t39025\t\"Brown County, OH\"\t39015\n\"Clermont County, OH\"\t39025\t\"Clermont County, OH\"\t39025\n\"Clermont County, OH
